vi "MilanHW3.vi"() -> ()   [LabVIEW 2020]
uses:
  <vilib>/Instr/_visa.llb/VISA Configure Serial Port (Instr).vi
panel:
  in  "Certainty":string
  in  "K":i32=5
  in  "Change K":bool
  out "new picture":picture
  out "Predictor":bool
  out "Z":dbl format="%#_13g"
  out "Y":dbl format="%#_13g"
  in  "Train_Deploy_Switch":bool
  in  "VISA resource name":refnum<visa-resource-name>
  in  "Done":bool
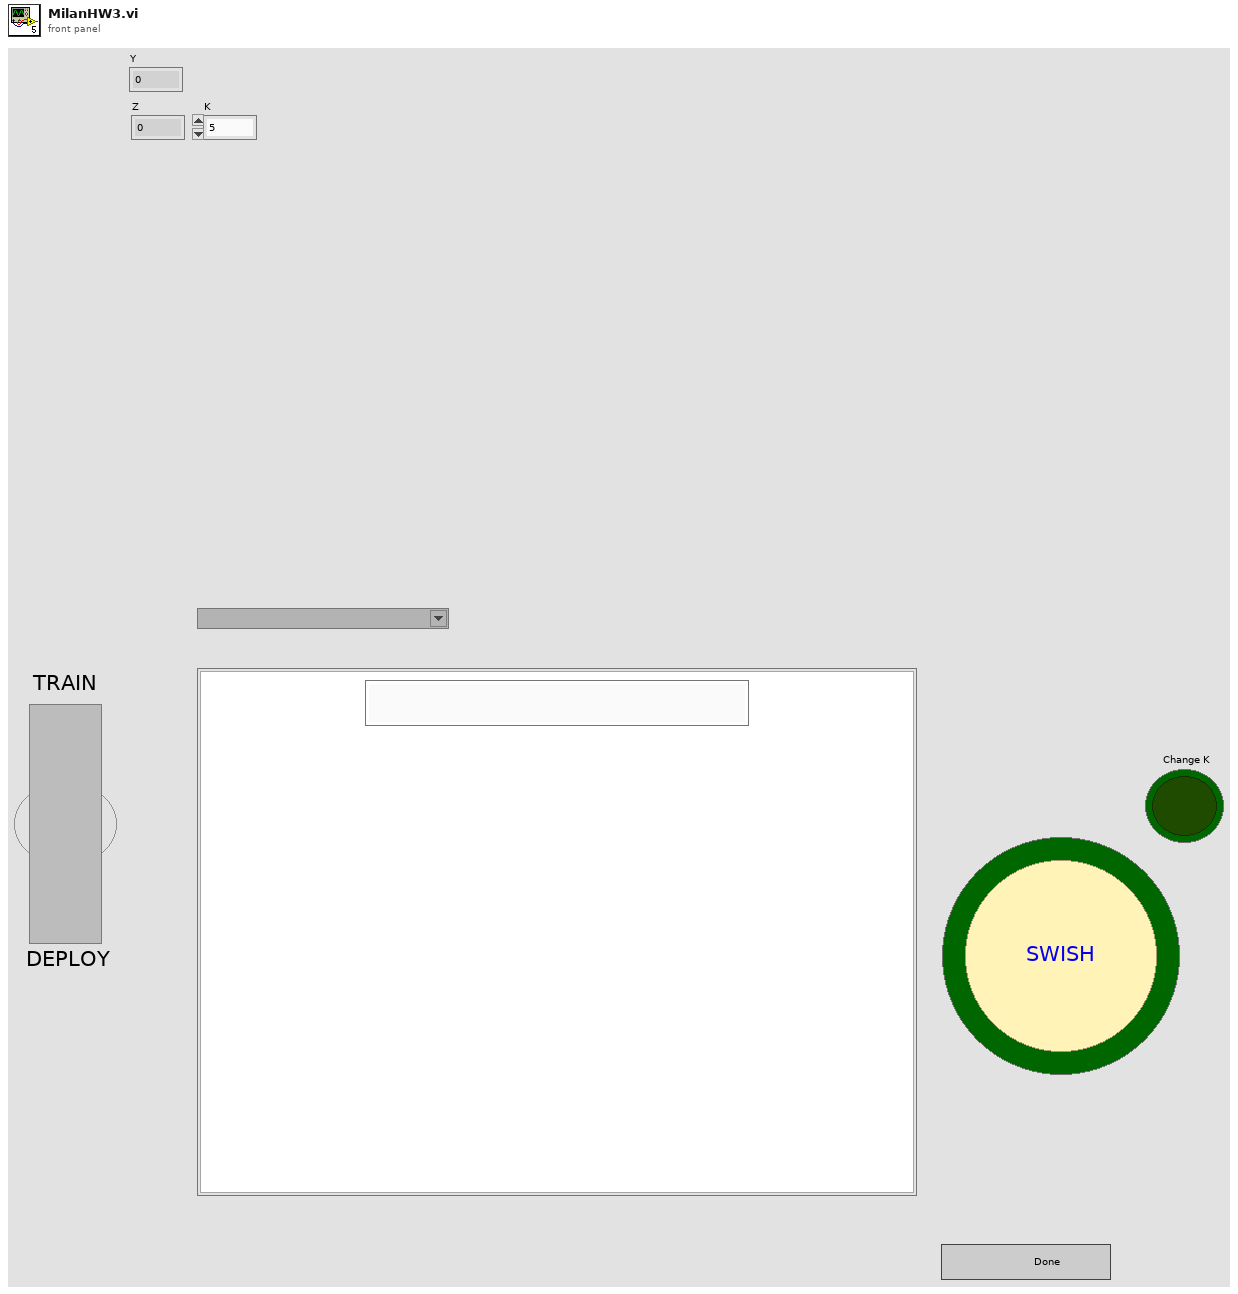
[diagram p1: front panel]
types:
  T1 = enum16{"Left Button", "Center Button", "Right Button", "Window Close"}
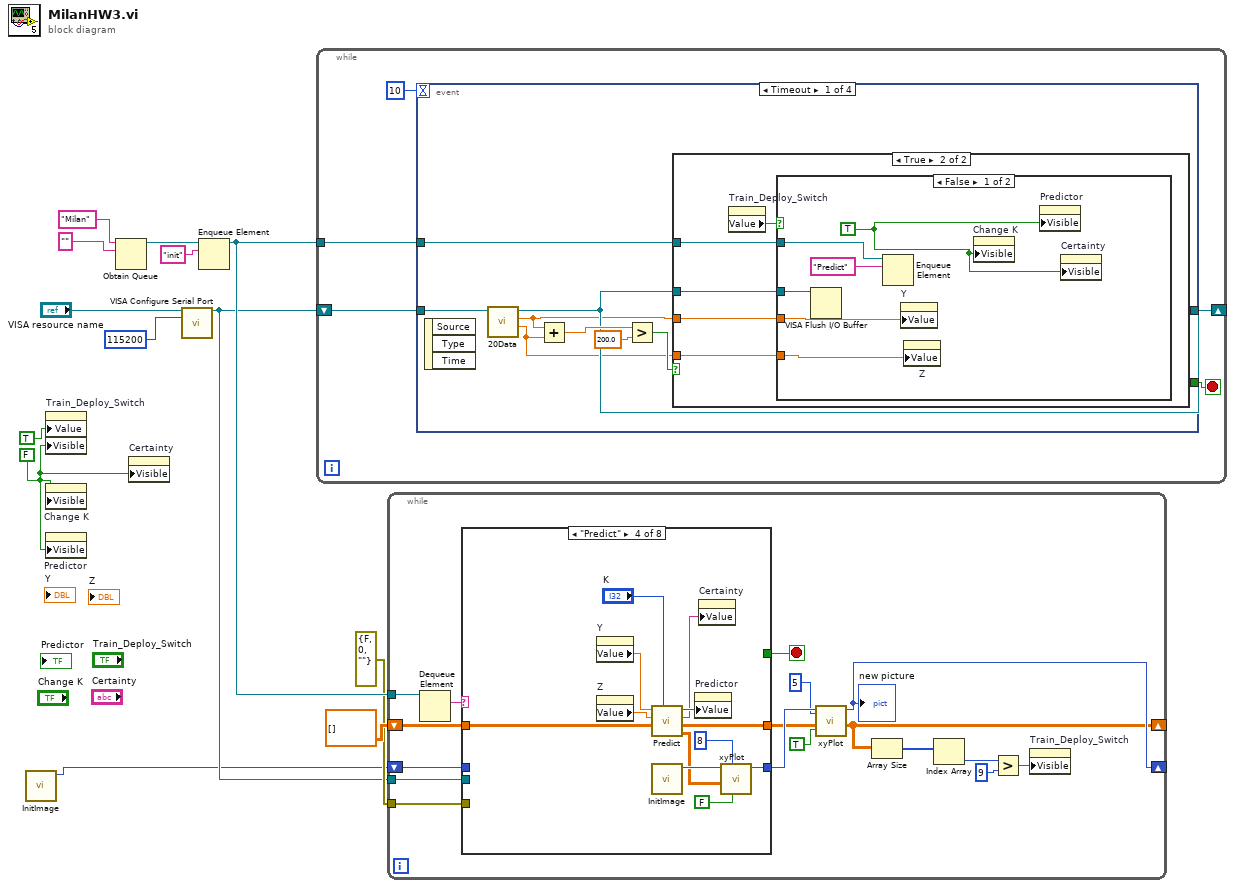
[diagram p0: block diagram]
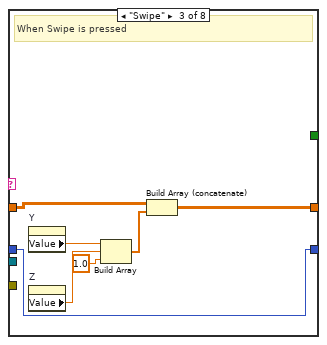
[diagram p4: hidden frame]
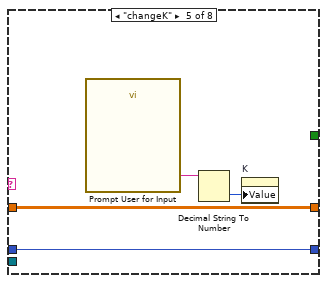
[diagram p5: hidden frame]
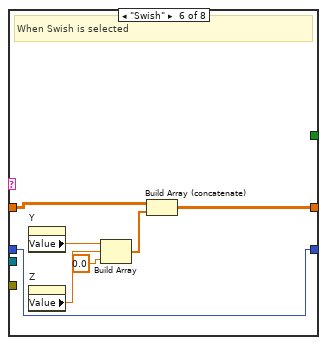
[diagram p6: hidden frame]
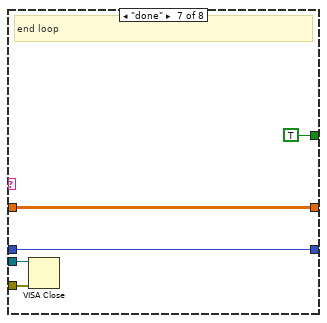
[diagram p7: hidden frame]
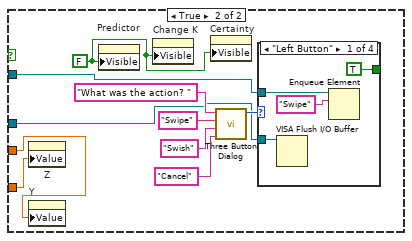
[diagram p10: hidden frame]
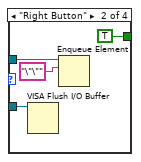
[diagram p11: hidden frame]
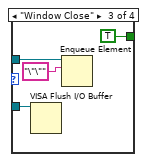
[diagram p12: hidden frame]
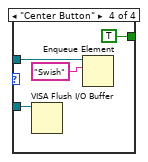
[diagram p13: hidden frame]
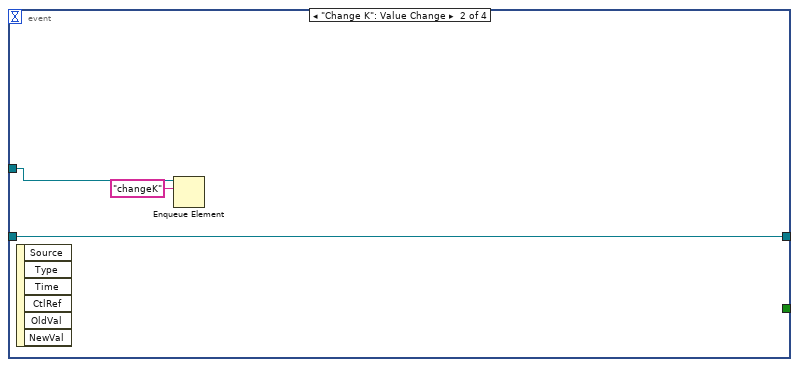
[diagram p14: hidden frame]
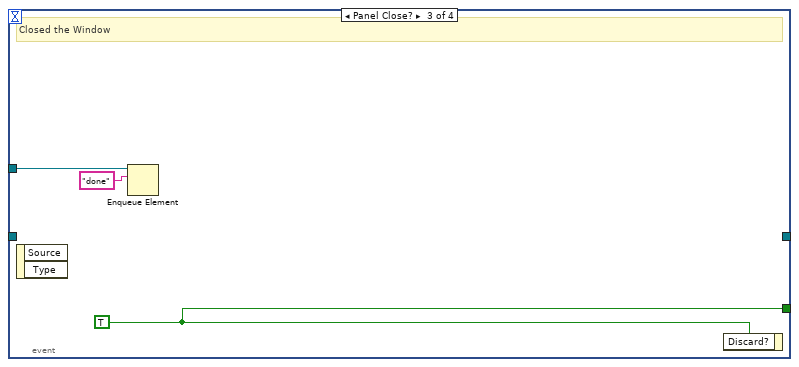
[diagram p15: hidden frame]
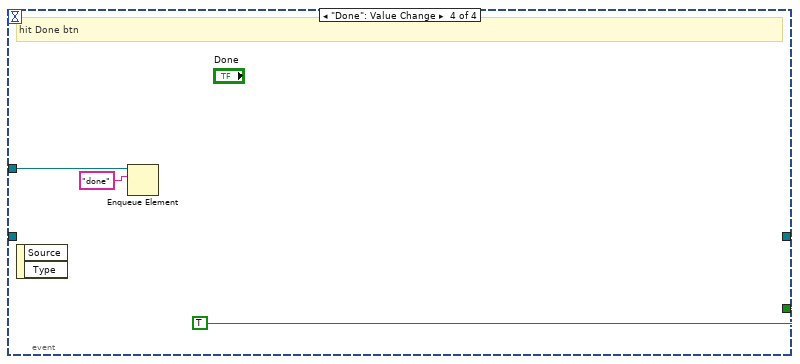
[diagram p16: hidden frame]
diagram:
  w1 = FALSE ("Visible")
  n1 = call "InitImage.vi"() -> ("new picture"=w2:picture)  [unwired: 11 in]
  n2 = property on="Train_Deploy_Switch" class="Bool (strict)"("Value"=TRUE ("Train_Deploy_Switch"), "Visible"=w1) -> ()  [unwired: 2 in, 2 out]
  n3 = property on="Change K" class="Bool (strict)"("Visible"=w1) -> ()  [unwired: 2 in, 2 out]
  n4 = property on="Predictor" class="Bool (strict)"("Visible"=w1) -> ()  [unwired: 2 in, 2 out]
  n5 = Obtain Queue(name (unnamed)="Milan", element data type="") -> (queue out=w13:refnum<queue>)  [unwired: 3 in, 2 out]
  n6 = property on="Certainty" class="Str"("Visible"=w1) -> ()  [unwired: 2 in, 2 out]
  n7 = call-poly "VISA Configure Serial Port"("VISA resource name"="VISA resource name", "baud rate (9600)"=u32 115200) -> ("VISA resource name out"=w4:refnum<visa-resource-name>)  [unwired: 12 in, 1 out]
  n8 = Enqueue Element(queue=w13, element="init") -> (queue out=w9:refnum<queue>)  [unwired: 2 in, 2 out]
  n9 = while {
    tunnel: w9 -> [w18]
    shift-right: [w14] -> _
    shift-left: w4 -> [w15]
    stop <- w17 stop-if-true
    n10 = event shown="[0] Timeout" {
      selector: _ -> [_ _ _ _]
      dyn-events: _ -> [_ _ _ _]
      timeout: 10 -> [_ _ _ _]
      tunnel: w18 -> [w25 w66 w68 w71]
      tunnel: [_ _ w67 TRUE ("Discard?")] -> w17
      tunnel: w15 -> [w24 w64 _ _]
      tunnel: [w21 w64 _ _] -> w14
      event Timeout {
        n11 = event-data() -> ()  [unwired: 1 in, 3 out]
        n12 = call "20Data.vi"("VISA resource name"=w24) -> ("Mean Z"=w19:dbl, "Mean Y"=w20:dbl, "VISA Refnum  out"=w21:refnum<visa-resource-name>)  [unwired: 7 in, 1 out]
        n13 = Add(x=w20, y=w19) -> (x+y=w23:dbl)
        n14 = Greater?(x=w23, y=200.0) -> (0:w22:bool)
        n15 = case shown="True" w22 {
          tunnel: w25 -> [_ w27]
          tunnel: w21 -> [_ w30]
          tunnel: w20 -> [_ w29]
          tunnel: w19 -> [_ w28]
          frame False {
          }
          frame True {
            n16 = property on="Train_Deploy_Switch" class="Bool (strict)"() -> ("Value"=w31:bool)  [unwired: 2 in, 2 out]
            n17 = case shown="False" w31 {
              tunnel: w27 -> [w37 w42]
              tunnel: w30 -> [w35 w41]
              tunnel: w29 -> [w33 w40]
              tunnel: w28 -> [w34 w39]
              frame False {
                w32 = TRUE ("Visible")
                n18 = VISA Flush I/O Buffer(VISA resource name=w35) -> ()  [unwired: 2 in, 2 out]
                n19 = Enqueue Element(queue=w37, element="Predict") -> ()  [unwired: 2 in, 3 out]
                n20 = property on="Y" class="DigNum (strict)"("Value"=w33) -> ()  [unwired: 2 in, 2 out]
                n21 = property on="Z" class="DigNum (strict)"("Value"=w34) -> ()  [unwired: 2 in, 2 out]
                n22 = property on="Change K" class="Bool (strict)"("Visible"=w32) -> ()  [unwired: 2 in, 2 out]
                n23 = property on="Predictor" class="Bool (strict)"("Visible"=w32) -> ()  [unwired: 2 in, 2 out]
                n24 = property on="Certainty" class="Str"("Visible"=w32) -> ()  [unwired: 2 in, 2 out]
              }
              frame True {
                w38 = FALSE ("Visible")
                n25 = property on="Z" class="DigNum (strict)"("Value"=w39) -> ()  [unwired: 2 in, 2 out]
                n26 = property on="Y" class="DigNum (strict)"("Value"=w40) -> ()  [unwired: 2 in, 2 out]
                n27 = property on="Predictor" class="Bool (strict)"("Visible"=w38) -> ()  [unwired: 2 in, 2 out]
                n28 = property on="Change K" class="Bool (strict)"("Visible"=w38) -> ()  [unwired: 2 in, 2 out]
                n29 = property on="Certainty" class="Str"("Visible"=w38) -> ()  [unwired: 2 in, 2 out]
                n30 = call <vilib>:"Three Button Dialog.vi"("Right Button Text (\"Cancel\")"="Cancel" ("Right Button Text (\"Cancel\")"), "Center Button Text (\"No\")"="Swish" ("Center Button Text (\"No\")"), "Left Button Text (\"Yes\")"="Swipe" ("Left Button Text (\"Yes\")"), "message"="What was the action? ") -> ("Which Button?"=w43:T1)  [unwired: 7 in]
                n31 = case shown="\"Left Button\"" w43 {
                  tunnel: w42 -> [w50 w54 w58 w62]
                  tunnel: [TRUE ("Flag") TRUE ("Flag") TRUE ("Flag") TRUE ("Boolean")] -> _
                  tunnel: w41 -> [w48 w52 w56 w60]
                  frame "Left Button" {
                    n32 = VISA Flush I/O Buffer(VISA resource name=w48) -> ()  [unwired: 2 in, 2 out]
                    n33 = Enqueue Element(queue=w50, element="Swipe") -> ()  [unwired: 2 in, 3 out]
                  }
                  frame "Right Button" {
                    n34 = VISA Flush I/O Buffer(VISA resource name=w52) -> ()  [unwired: 2 in, 2 out]
                    n35 = Enqueue Element(queue=w54, element="\"\"") -> ()  [unwired: 2 in, 3 out]
                  }
                  frame "Window Close" {
                    n36 = VISA Flush I/O Buffer(VISA resource name=w56) -> ()  [unwired: 2 in, 2 out]
                    n37 = Enqueue Element(queue=w58, element="\"\"") -> ()  [unwired: 2 in, 3 out]
                  }
                  frame "Center Button" {
                    n38 = VISA Flush I/O Buffer(VISA resource name=w60) -> ()  [unwired: 2 in, 2 out]
                    n39 = Enqueue Element(queue=w62, element="Swish") -> ()  [unwired: 2 in, 3 out]
                  }
                }
              }
            }
          }
        }
      }
      event "Change K": Value Change {
        n40 = event-data() -> ()  [unwired: 1 in, 6 out]
        n41 = Enqueue Element(queue=w66, element="changeK") -> ()  [unwired: 2 in, 3 out]
      }
      event Panel Close? {
        w67 = TRUE ("Discard?")
        # "Closed the Window"
        n42 = event-data() -> ()  [unwired: 1 in, 2 out]
        n43 = Enqueue Element(queue=w68, element="done") -> ()  [unwired: 2 in, 3 out]
        n44 = event-data("Discard?"=w67) -> ()  [unwired: 1 in, 1 out]
      }
      event "Done": Value Change {
        # "hit Done btn"
        n45 = event-data() -> ()  [unwired: 1 in, 2 out]
        n46 = Enqueue Element(queue=w71, element="done") -> ()  [unwired: 2 in, 3 out]
      }
    }
  }
  n47 = while {
    tunnel: w9 -> [w89]
    shift-right: [w75] -> _
    shift-left: dbl[][] [] -> [w86]
    tunnel: errorcluster {"status"=FALSE, "code"=0, "source"=""} ("error out") -> [w85]
    tunnel: w4 -> [w80]
    shift-right: [w79] -> _
    shift-left: w2 -> [w78]
    stop <- w87 stop-if-true
    n48 = Dequeue Element(queue=w89) -> (element=w88:string)  [unwired: 2 in, 3 out]
    n49 = case shown="\"Predict\"" w88 {
      tunnel: [_ _ _ _ _ _ TRUE ("Discard?") _] -> w87
      tunnel: w86 -> [w91 w93 w100 w112 w116 w123 w127 w130]
      tunnel: [w91 w93 w99 w107 w116 w122 w127 w130] -> w76
      tunnel: w85 -> [_ _ _ _ _ _ w126 _]
      tunnel: w80 -> [_ _ _ _ _ _ w125 _]
      tunnel: w78 -> [w90 w92 w96 _ w115 w119 w124 w129]
      tunnel: [w90 w92 w96 w103 w115 w119 w124 w129] -> w77
      frame Default {
      }
      frame "init" {
        # "Initialize things here"
      }
      frame "Swipe" {
        # "When Swipe is pressed"
        n50 = property on="Y" class="DigNum (strict)"() -> ("Value"=w95:dbl)  [unwired: 2 in, 2 out]
        n51 = property on="Z" class="DigNum (strict)"() -> ("Value"=w94:dbl)  [unwired: 2 in, 2 out]
        n52 = Build Array(w95, w94, 1.0 ("element")) -> (w98:dbl[])
        n53 = Build Array (concatenate)(w100, w98) -> (w99:dbl[][])
      }
      frame "Predict" {
        n54 = property on="Y" class="DigNum (strict)"() -> ("Value"=w110:dbl)  [unwired: 2 in, 2 out]
        n55 = property on="Z" class="DigNum (strict)"() -> ("Value"=w109:dbl)  [unwired: 2 in, 2 out]
        n56 = call "Predict.vi"("K"="K", "Array In"=w112, "Z"=w109, "Y"=w110) -> ("Sorted Data points"=w104:dbl[][], "Arrary Out"=w107:dbl[][], "concatenated string"=w101:string, "Boolean"=w111:bool)  [unwired: 4 in]
        n57 = call "InitImage.vi"() -> ("new picture"=w105:picture)  [unwired: 11 in]
        n58 = property on="Predictor" class="Bool (strict)"("Value"=w111) -> ()  [unwired: 2 in, 2 out]
        n59 = property on="Certainty" class="Str"("Value"=w101) -> ()  [unwired: 2 in, 2 out]
        n60 = call "xyPlot.vi"("fill?(F)"=FALSE, "radius"=i16 8, "Array In"=w104, "new picture in"=w105) -> ("new picture out"=w103:picture)  [unwired: 6 in, 1 out]
      }
      frame "changeK" {
        n61 = call "Prompt User for Input"() -> ("K"=w114:string)  [unwired: 17 in, 2 out]
        n62 = Decimal String To Number(string=w114) -> (number=w113:i32)  [unwired: 2 in, 1 out]
        n63 = property on="K" class="DigNum (strict)"("Value"=w113) -> ()  [unwired: 2 in, 2 out]
      }
      frame "Swish" {
        # "When Swish is selected"
        n64 = property on="Y" class="DigNum (strict)"() -> ("Value"=w118:dbl)  [unwired: 2 in, 2 out]
        n65 = property on="Z" class="DigNum (strict)"() -> ("Value"=w117:dbl)  [unwired: 2 in, 2 out]
        n66 = Build Array(w118, w117, 0.0 ("element")) -> (w121:dbl[])
        n67 = Build Array (concatenate)(w123, w121) -> (w122:dbl[][])
      }
      frame "done" {
        # "end loop"
        n68 = VISA Close(VISA resource name=w125, error in (no error)=w126) -> ()  [unwired: 1 out]
      }
      frame "" {
      }
    }
    n69 = call "xyPlot.vi"("fill?(F)"=TRUE, "radius"=i16 5, "Array In"=w76, "new picture in"=w77) -> ("Array Out"=w75:dbl[][], "new picture out"=w79:picture)  [unwired: 6 in]
    "new picture" <- w79
    n70 = Array Size(array=w75) -> (size(s)=w84:i32[])
    n71 = Index Array(array=w84) -> (element=w83:i32)  [unwired: 1 in]
    n72 = Greater?(x=w83, y=9) -> (0:w81:bool)
    n73 = property on="Train_Deploy_Switch" class="Bool (strict)"("Visible"=w81) -> ()  [unwired: 2 in, 2 out]
  }
